vi "Prepare Paths For Expiration Check.vi"(0 "Vector Path Group in":refnum<class "Vector Path Group.lvclass">, 5 "TSM Context":T1, 11 "error in (no error)":errorcluster) -> (4 "Vector Path Group out":refnum<class "Vector Path Group.lvclass">, 15 "error out":errorcluster)   [LabVIEW 2023, in "RFFixtureCharact.Public.lvlib" / "Vector Path Group.lvclass"]
uses:
  Vector Path Group.lvclass
  C:/rfcal/AuxTools/STSRFFixtureCharactUtility/Source/Code Modules/Common/Base Classes/Path Group/Path Group.lvclass
  <vilib>/NI_TestStand_SemiconductorModule/NI_TestStand_Semiconductor_Module.lvlibp/PinMap/General/SemiconductorModuleContext.ctl
  Vector Path/Vector Path.lvclass
  C:/rfcal/AuxTools/STSRFFixtureCharactUtility/Source/Code Modules/Common/Base Classes/Path/Path.lvclass
  Charact Result Accessor/Vector/Vector Charact Result Accessor.lvclass
  C:/rfcal/AuxTools/STSRFFixtureCharactUtility/Source/Code Modules/Fixture/Public/Charact Result Accessor/Base/Charact Result Accessor.lvclass
  C:/rfcal/AuxTools/STSRFFixtureCharactUtility/Source/Code Modules/Common/Result Accessor/Result Accessor.lvclass
  Common/Base Classes/Path/Path.lvclass/Path.ctl
  Common/Base Classes/Path/Properties/Read Interval.vi
  Common/Base Classes/Path/Path.lvclass
  Common/Base Classes/Path Group/Path Group.lvclass
  <vilib>/NI_TestStand_SemiconductorModule/NI_TestStand_Semiconductor_Module.lvlibp
  Common/RFCalAndFixtureCharact.Common.lvlib
  <vilib>/addons/_RFCalAndCharactDatabase/NI_RFCalAndCharact_Database_API.lvlibp/Characterization/Characterization.lvlib
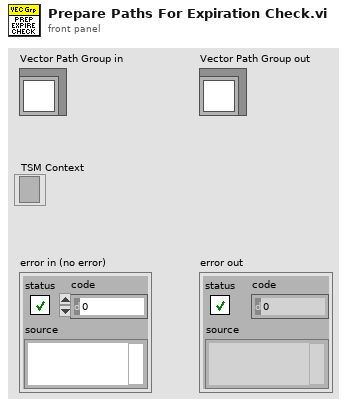
[diagram p1: front panel]
types:
  T1 = typedef "NI_TestStand_Semiconductor_Module.lvlibp/SemiconductorModuleContext.ctl" = refnum<k7>
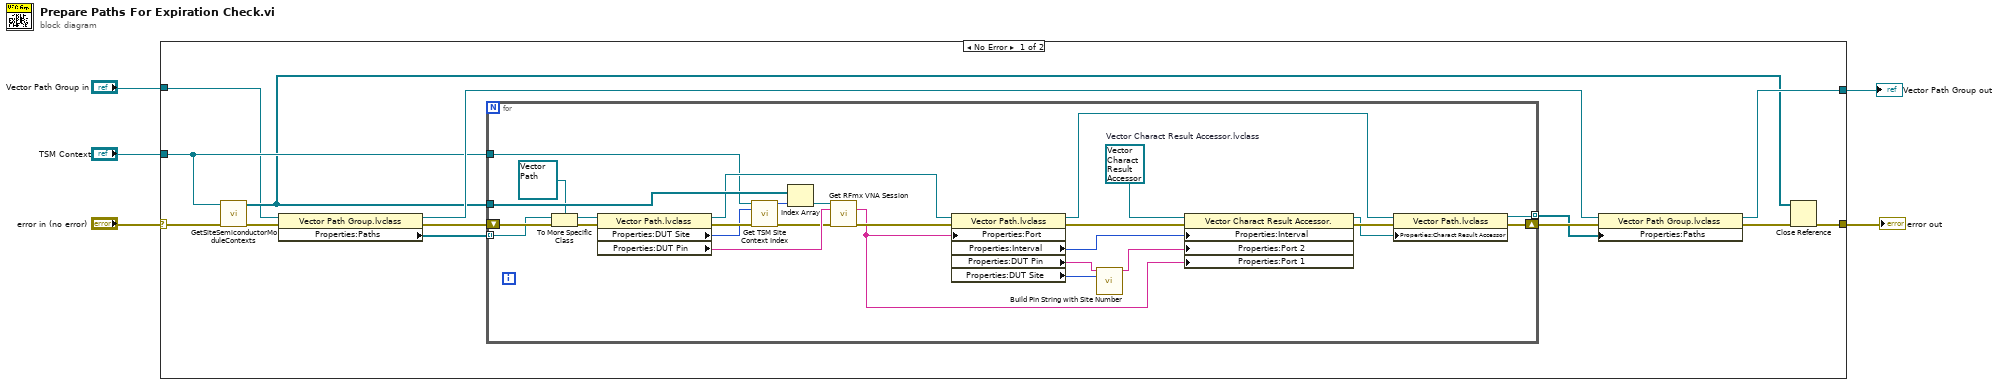
[diagram p0: block diagram]
diagram:
  n1 = case shown="No Error" "error in (no error)" {
    selector: "error in (no error)" -> [w11 w47]
    tunnel: "TSM Context" -> [w13 _]
    tunnel: "Vector Path Group in" -> [w6 w46]
    tunnel: [w14 w47] -> w1
    tunnel: [w15 w46] -> w2
    frame No Error {
      n2 = call <vilib>:"GetSiteSemiconductorModuleContexts.vi"("error in (no error)"=w11, "Semiconductor Module Context"=w13) -> ("error out"=w17:errorcluster, "Site Semiconductor Module Contexts"=w9:T1[])  [unwired: 8 in]
      n3 = property class="Vector Path Group.lvclass"(reference=w6, error in=w17) -> (reference out=w16:refnum<class "Vector Path Group.lvclass">, error out=w18:errorcluster, "Properties:Paths"=w10:refnum<class "Path.lvclass">[])
      n4 = for {
        tunnel: w9 -> [w45]
        tunnel: w10 -> [w39] mode=indexing
        tunnel: [w27] -> w7 mode=indexing
        tunnel: w13 -> [w33]
        shift-right: [w28] -> w8
        shift-left: w18 -> [w41]
        w22 = refnum<class "Vector Charact Result Accessor.lvclass"> refnum  # Vector Charact Result Accessor.lvclass
        n5 = To More Specific Class(target class=refnum<class "Vector Path.lvclass"> refnum ("STS Vector Fixture Charact.lvlib:Vector Path.lvclass"), reference=w39, error in=w41) -> (specific class reference=w38:refnum<class "Vector Path.lvclass">, error out=w40:errorcluster)
        n6 = property class="Vector Path.lvclass"(reference=w38, error in=w40) -> (reference out=w42:refnum<class "Vector Path.lvclass">, error out=w43:errorcluster, "Properties:DUT Site"=w35:i32, "Properties:DUT Pin"=w37:string)
        n7 = call "Get TSM Site Context Index.vi"("Semiconductor Module Context"=w33, "Site Number"=w35, "error in (no error)"=w43) -> ("index of Site TSM Context"=w34:i32, "error out"=w36:errorcluster)  [unwired: 11 in]
        n8 = Index Array(array=w45, index=w34) -> (element=w44:T1)
        n9 = call "Get RFmx VNA Session.vi"("TSM Context"=w44, "Pin"=w37, "error in"=w36) -> ("Port"=w23:string, "error out"=w32:errorcluster)  [unwired: 10 in, 1 out]
        n10 = property class="Vector Path.lvclass"(reference=w42, error in=w32, "Properties:Port"=w23) -> (reference out=w26:refnum<class "Vector Path.lvclass">, error out=w21:errorcluster, "Properties:Interval"=w19:i32, "Properties:DUT Pin"=w25:string, "Properties:DUT Site"=w24:i32)
        n11 = call <vilib>:"Build Pin String with Site Number.vi"("Pin Name"=w25, "Site Number"=w24) -> ("Pin String"=w20:string)  [unwired: 13 in]
        n12 = property class="Vector Charact Result Accessor."(reference=w22, error in=w21, "Properties:Interval"=w19, "Properties:Port 2"=w20, "Properties:Port 1"=w23) -> (reference out=w29:refnum<class "Vector Charact Result Accessor.lvclass">, error out=w30:errorcluster)
        n13 = property class="Vector Path.lvclass"(reference=w26, error in=w30, "Properties:Charact Result Accessor"=w29) -> (reference out=w27:refnum<class "Vector Path.lvclass">, error out=w28:errorcluster)
      }
      n14 = property class="Vector Path Group.lvclass"(reference=w16, error in=w8, "Properties:Paths"=w7) -> (reference out=w15:refnum<class "Vector Path Group.lvclass">, error out=w12:errorcluster)
      n15 = Close Reference(reference=w9, error in (no error)=w12) -> (error out=w14:errorcluster)
    }
    frame Error {
    }
  }
  "error out" <- w1
  "Vector Path Group out" <- w2
